vi "loadLutFile.vi"(0 "connection ID":i32, 5 "axis":i32, 9 "Path to LUT file":path, 11 "error in":errorcluster) -> (4 "connection ID":i32, 6 "axis_out":i32, 15 "error out":errorcluster)   [LabVIEW 2016]
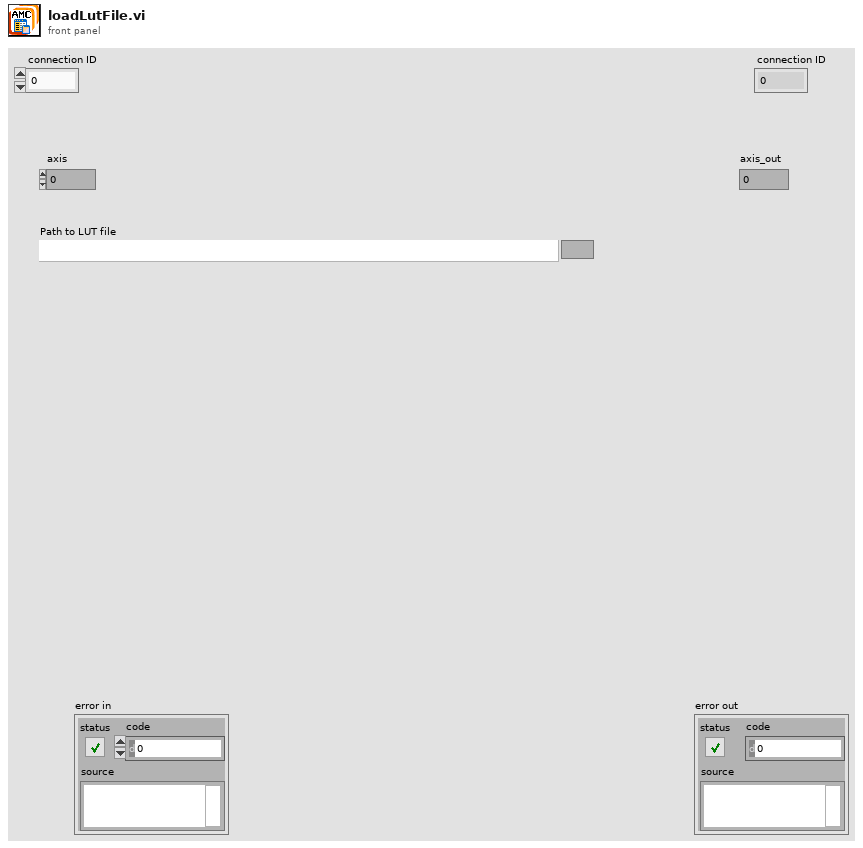
[diagram p1: front panel]
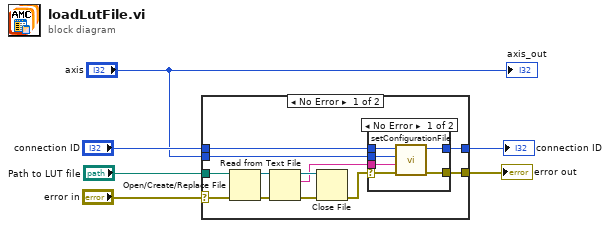
[diagram p0: block diagram]
diagram:
  n1 = case shown="No Error" "error in" {
    selector: "error in" -> [w9 w28]
    tunnel: [w10 w28] -> w6
    tunnel: [w17 w27] -> w5
    tunnel: "connection ID" -> [w18 w27]
    tunnel: "axis" -> [w12 _]
    tunnel: "Path to LUT file" -> [w8 _]
    frame No Error {
      n2 = Open/Create/Replace File(file path (use dialog)=w8, error in=w9) -> (refnum out=w7:refnum<file>, error out=w16:errorcluster)  [unwired: 4 in, 1 out]
      n3 = Read from Text File(file (use dialog)=w7, error in=w16) -> (refnum out=w14:refnum<file>, text=w13:string, error out=w15:errorcluster)  [unwired: 2 in, 1 out]
      n4 = Close File(refnum=w14, error in=w15) -> (error out=w11:errorcluster)  [unwired: 1 out]
      n5 = case shown="No Error" w11 {
        selector: w11 -> [w20 w26]
        tunnel: w18 -> [w24 w25]
        tunnel: [w23 w25] -> w17
        tunnel: w13 -> [w22 _]
        tunnel: w12 -> [w21 _]
        tunnel: [w19 w26] -> w10
        frame No Error {
          n6 = call "setConfigurationFile.vi"("error in"=w20, "content"=w22, "axis"=w21, "connection ID"=w24) -> ("error out"=w19:errorcluster, "connection ID"=w23:i32)  [unwired: 5 in, 1 out]
        }
        frame Error {
        }
      }
    }
    frame Error {
    }
  }
  "error out" <- w6
  "connection ID" <- w5
  "axis_out" <- "axis"
